vi "Discovery.vi"(8 "error in (no error)":errorcluster, 10 "Device Name Or Device Address":string, 11 "BT in":refnum<class "BT.lvclass">) -> (0 "error out":errorcluster, 3 "BT out":refnum<class "BT.lvclass">)   [LabVIEW 2014, in "BT.lvlib" / "BT.lvclass"]
uses:
  BT.lvclass
  BT.lvclass/BT.ctl
  C:/Users/yang/Desktop/BT Connect/InTheHand.Net.Personal.dll
  BT Connect/InTheHand.Net.Personal.dll
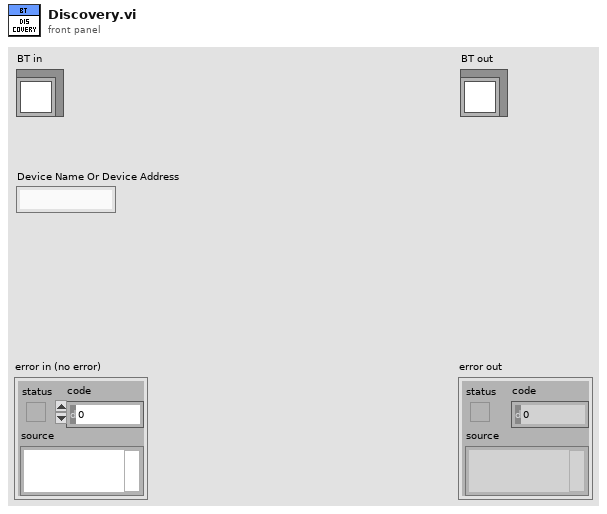
[diagram p1: front panel]
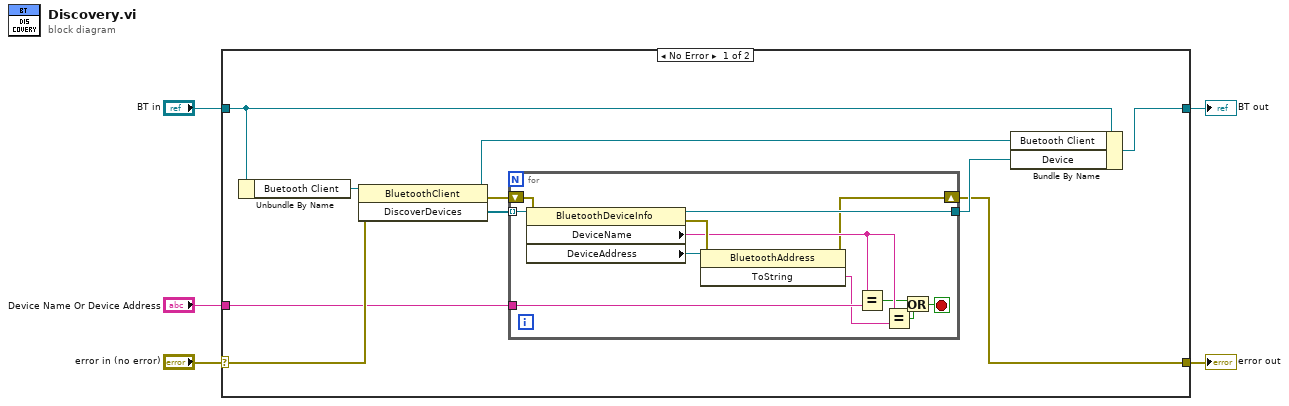
[diagram p0: block diagram]
diagram:
  n1 = case shown="No Error" "error in (no error)" {
    selector: "error in (no error)" -> [w14 w29]
    tunnel: [w6 w29] -> w4
    tunnel: [w7 w28] -> w2
    tunnel: "BT in" -> [w8 w28]
    tunnel: "Device Name Or Device Address" -> [w12 _]
    frame No Error {
      n2 = Unbundle By Name(w8) -> ("Buetooth Client"=w15:refnum<k24>)
      n3 = invoke class="BluetoothClient" method="DiscoverDevices"(reference=w15, error in=w14) -> (reference out=w10:refnum<k24>, error out=w11:errorcluster, "DiscoverDevices"=w13:refnum<k24>[])  [unwired: 1 in]
      n4 = for {
        tunnel: w13 -> [w27] mode=indexing
        tunnel: w12 -> [w23]
        tunnel: [w17] -> w9
        shift-right: [w16] -> w6
        shift-left: w11 -> [w26]
        stop <- w18 stop-if-true
        n5 = property class="BluetoothDeviceInfo"(reference=w27, error in=w26) -> (reference out=w17:refnum<k24>, error out=w24:errorcluster, "DeviceName"=w22:string, "DeviceAddress"=w25:refnum<k24>)
        n6 = invoke class="BluetoothAddress" method="ToString"(reference=w25, error in=w24) -> (error out=w16:errorcluster, "ToString"=w21:string)  [unwired: 1 in, 1 out]
        n7 = Equal?(x=w22, y=w23) -> (x = y?=w20:bool)
        n8 = Equal?(x=w22, y=w21) -> (x = y?=w19:bool)
        n9 = Or(x=w20, y=w19) -> (x .or. y?=w18:bool)
      }
      n10 = Bundle By Name(cluster=w8, "Buetooth Client"=w10, "Device"=w9) -> (w7:refnum<class "BT.lvclass">)
    }
    frame Error {
    }
  }
  "error out" <- w4
  "BT out" <- w2
